vi "Ex2_Grafica y Guarda.vi"(8 "error in (no error)":errorcluster, 10 "Señales Procesadas":T1, 11 "Señales":T2) -> (0 "error out":errorcluster, 2 "Señales Procesadas Digitales":dynamicdata(graph), 3 "Señales Procesadas Ang":dynamicdata(graph))   [LabVIEW 2020]
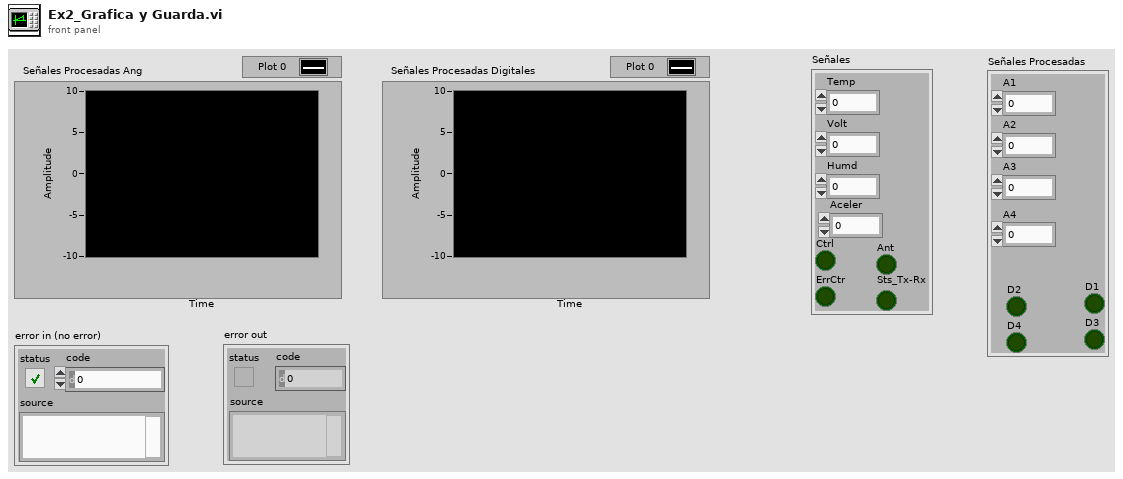
[diagram p1: front panel]
types:
  T1 = cluster{"D1":bool, "D3":bool, "A1":dbl, "A2":dbl, "A3":dbl, "D2":bool, "D4":bool, "A4":dbl}
  T2 = cluster{"Temp":dbl, "Volt":dbl, "Humd":dbl, "Ant":bool, "Ctrl":bool, "ErrCtr":bool, "Aceler":dbl, "Sts_Tx-Rx":bool}
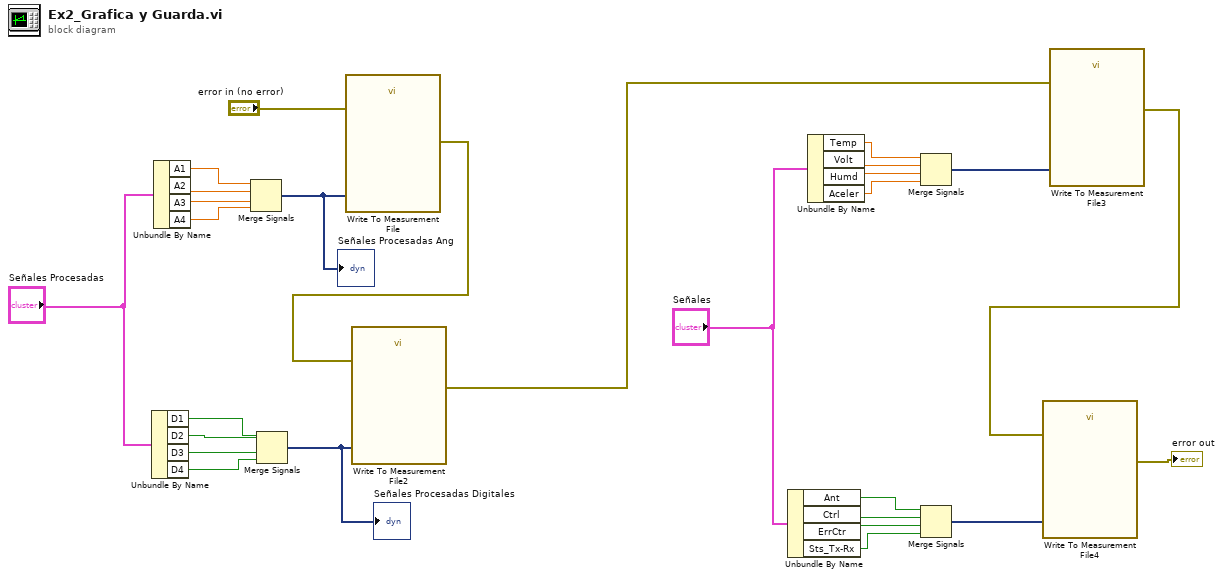
[diagram p0: block diagram]
diagram:
  n1 = Unbundle By Name("Señales Procesadas") -> ("D1"=w21:bool, "D2"=w20:bool, "D3"=w19:bool, "D4"=w17:bool)
  n2 = Unbundle By Name("Señales Procesadas") -> ("A1"=w26:dbl, "A2"=w25:dbl, "A3"=w24:dbl, "A4"=w23:dbl)
  n3 = Merge Signals(w26, w25, w24, w23) -> (w22:dynamicdata)
  "Señales Procesadas Ang" <- w22
  n4 = Merge Signals(w21, w20, w19, w17) -> (w18:dynamicdata)
  "Señales Procesadas Digitales" <- w18
  n5 = call "Write To Measurement File"("Signals"=w22, "error in (no error)"="error in (no error)") -> ("error out"=w6:errorcluster)  [unwired: 15 in, 2 out]
  n6 = call "Write To Measurement File2"("Signals"=w18, "error in (no error)"=w6) -> ("error out"=w5:errorcluster)  [unwired: 15 in, 2 out]
  n7 = Unbundle By Name("Señales") -> ("Ant"=w9:bool, "Ctrl"=w11:bool, "ErrCtr"=w10:bool, "Sts_Tx-Rx"=w1:bool)
  n8 = Unbundle By Name("Señales") -> ("Temp"=w15:dbl, "Volt"=w13:dbl, "Humd"=w12:dbl, "Aceler"=w14:dbl)
  n9 = Merge Signals(w15, w13, w12, w14) -> (w7:dynamicdata)
  n10 = Merge Signals(w9, w11, w10, w1) -> (w8:dynamicdata)
  n11 = call "Write To Measurement File3"("Signals"=w7, "error in (no error)"=w5) -> ("error out"=w4:errorcluster)  [unwired: 15 in, 2 out]
  n12 = call "Write To Measurement File4"("Signals"=w8, "error in (no error)"=w4) -> ("error out"=→"error out":errorcluster)  [unwired: 15 in, 2 out]
